vi "Configure Autozero State.vi"(8 "error in (no error)":errorcluster, 9 "Auto Zero State":bool, 10 "Function":u16(ring) items=["Voltage: DC", "Voltage: AC", "Current: DC", "Current: AC", "2W Resistance", "4W Resistance", "Diode", "Capacitance", "Temperature", "Continuity", "Frequency", "Period", "Ratio", "Digitize Voltage", "Digitize Current"], 11 "VISA resource name":refnum<visa-resource-name>) -> (0 "error out":errorcluster, 3 "VISA resource name out":refnum<visa-resource-name>)   [LabVIEW 2009, in "Keithley DMM7510.lvlib"]
doc: "Enables or disables the autozero function on the instrument. Enabling autozero optimizes the instrument for accuracy, while disabling optimizes for speed."
uses:
  Keithley DMM7510.lvlib
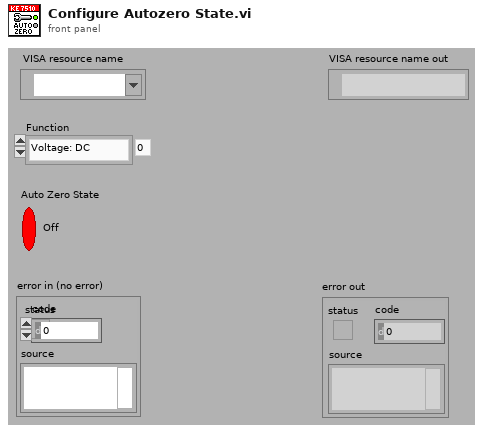
[diagram p1: front panel]
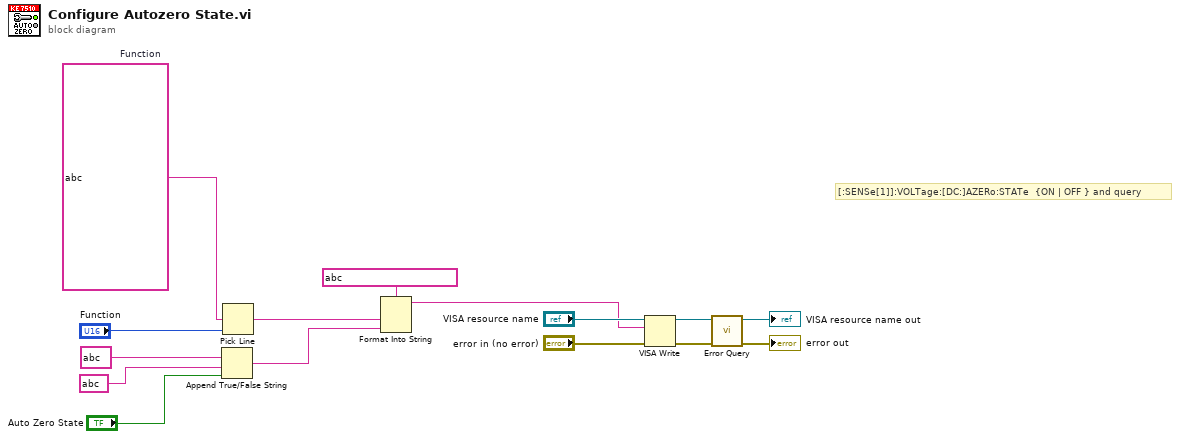
[diagram p0: block diagram]
diagram:
  w2 = string ?  # Function
  # "[:SENSe[1]]:VOLTage:[DC:]AZERo:STATe  {ON | OFF } and query"
  n1 = Append True/False String(1:"Auto Zero State", 2:string ? ("write buffer"), 3:string ? ("write buffer")) -> (0:w4:string)  [unwired: 1 in]
  n2 = Pick Line(multi-line string=w2, line index="Function") -> (output string=w8:string)  [unwired: 1 in]
  n3 = Format Into String(format string=string ? ("write buffer"), w8, w4) -> (resulting string=w3:string)  [unwired: 2 in, 1 out]
  n4 = VISA Write(VISA resource name="VISA resource name", write buffer=w3, error in (no error)="error in (no error)") -> (VISA resource name out=w11:refnum<visa-resource-name>, error out=w10:errorcluster)  [unwired: 1 out]
  n5 = call "Error Query.vi"("error in (no error)"=w10, "VISA resource name"=w11) -> ("error out"=→"error out":errorcluster, "VISA resource name out"=→"VISA resource name out":refnum<visa-resource-name>)  [unwired: 8 out]
